vi "Run.vi"(8 "error in (no error)":errorcluster, 11 "Opctics in":refnum<class "Opt_Selector.lvclass">) -> (0 "error out":errorcluster, 3 "Opt_Selector out":refnum<class "Opt_Selector.lvclass">)   [LabVIEW 2018, in "Opt_Selector.lvclass"]
uses:
  Opt_Selector.lvclass
  Optics.lvclass/Optics.ctl
  Optics.lvclass
  StateMachine/State Machine.lvclass
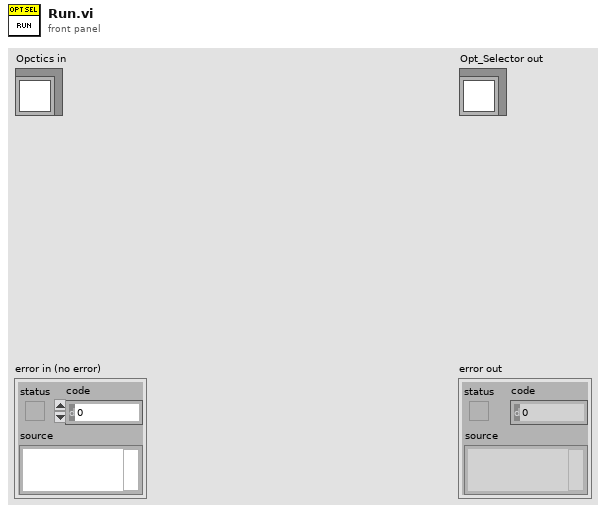
[diagram p1: front panel]
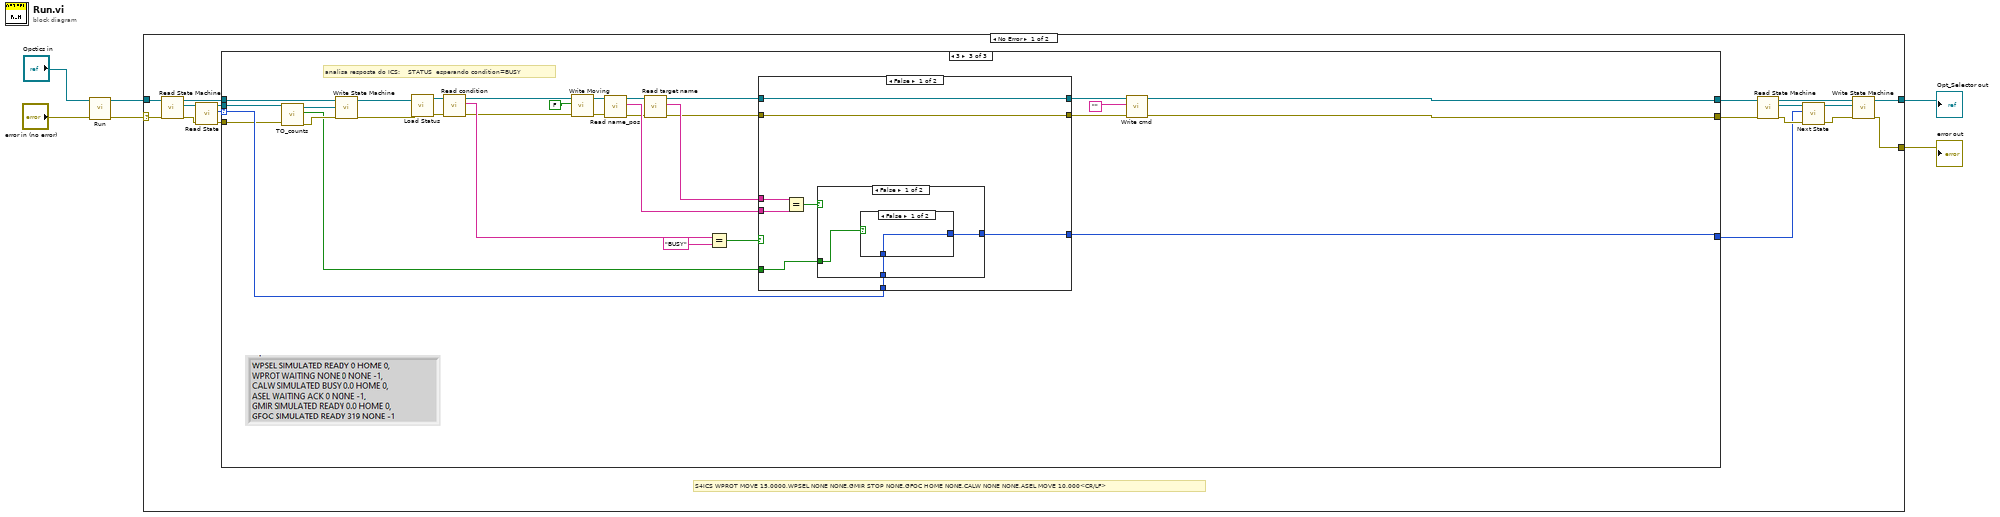
[diagram p0: block diagram]
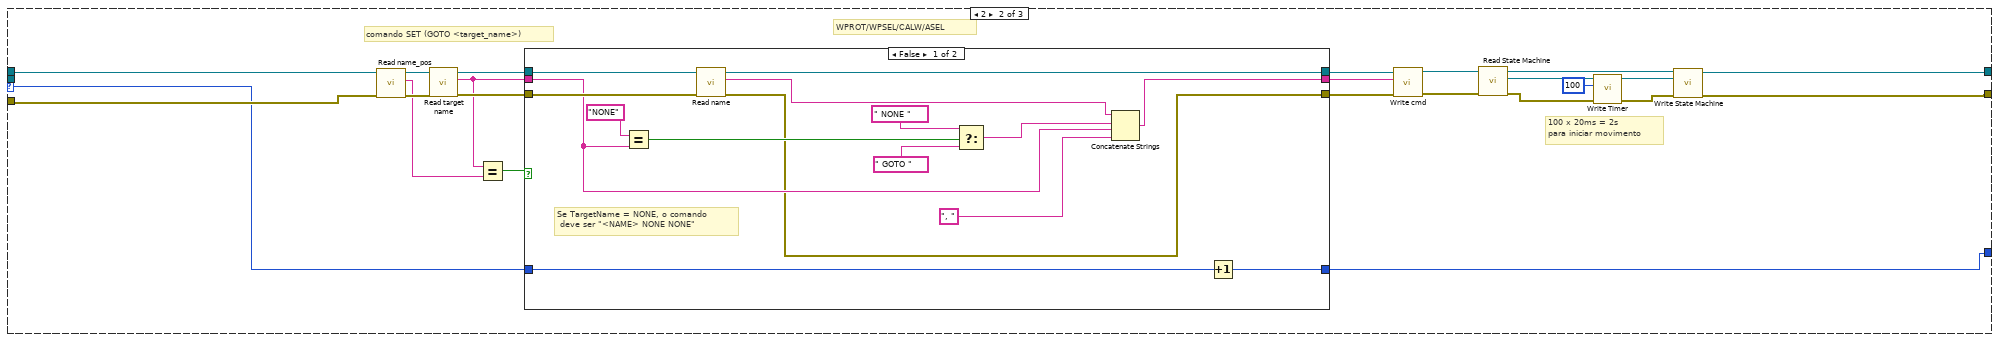
[diagram p3: hidden frame]
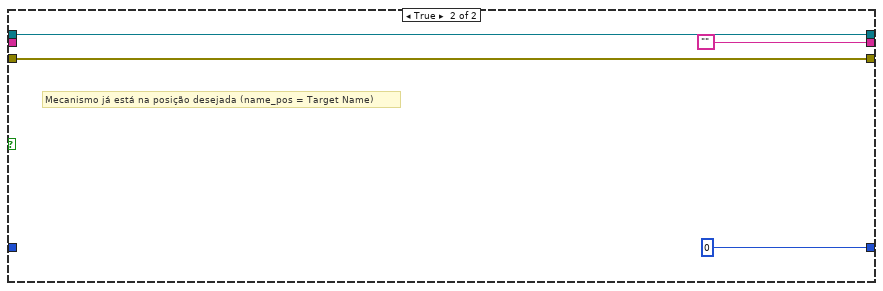
[diagram p4: hidden frame]
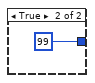
[diagram p5: hidden frame]
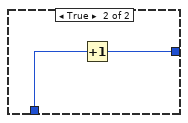
[diagram p6: hidden frame]
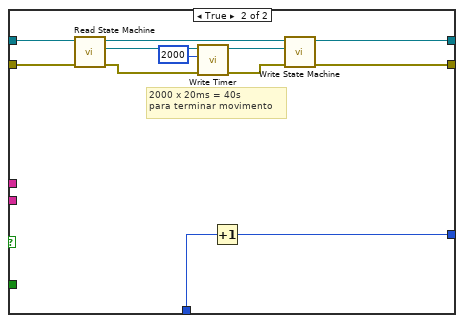
[diagram p7: hidden frame]
diagram:
  n1 = call-parent "Run.vi"("error in (no error)"="error in (no error)", "Opctics in"="Opctics in") -> ("error out"=w3:errorcluster, "Optics out"=w4:refnum<class "Opt_Selector.lvclass">)  [unwired: 8 in]
  n2 = case shown="No Error" w3 {
    selector: w3 -> [w23 w130]
    tunnel: [w8 w130] -> w1
    tunnel: [w13 w129] -> w2
    tunnel: w4 -> [w24 w129]
    frame No Error {
      # "S4ICS WPROT MOVE 15.0000,WPSEL NONE NONE,GMIR STOP NONE,GFOC HOME NONE,CALW NONE NONE,ASEL MOVE 10.000<CR/LF>"
      n3 = call-dynamic "Read State Machine.vi"("error in (no error)"=w23, "Device in"=w24) -> ("error out"=w20:errorcluster, "State Machine.lvclass"=w22:refnum<class "State Machine.lvclass">, "Device out"=w18:refnum<class "Opt_Selector.lvclass">)  [unwired: 7 in]
      n4 = call-dynamic "Read State.vi"("error in (no error)"=w20, "State Machine in"=w22) -> ("error out"=w19:errorcluster, "State"=w21:i32, "State Machine out"=w7:refnum<class "State Machine.lvclass">)  [unwired: 7 in]
      n5 = case shown="3" w21 {
        selector: w21 -> [w27 w45 w97]
        tunnel: w19 -> [w25 w48 w77]
        tunnel: [w25 w28 w99] -> w9
        tunnel: w18 -> [w26 w49 w80]
        tunnel: [w26 w29 w100] -> w16
        tunnel: [w27 w44 w98] -> w10
        tunnel: w7 -> [_ _ w76]
        frame Default {
        }
        frame 2 {
          # "100 x 20ms = 2s\npara iniciar movimento"
          # "WPROT/WPSEL/CALW/ASEL"
          # "comando SET (GOTO <target_name>)"
          n6 = call "Read name_pos.vi"("error in (no error)"=w48, "Optics in"=w49) -> ("error out"=w47:errorcluster, "name_pos"=w41:string, "Optics out"=w46:refnum<class "Opt_Selector.lvclass">)  [unwired: 7 in]
          n7 = call "Read target name.vi"("error in (no error)"=w47, "Optics in"=w46) -> ("error out"=w51:errorcluster, "target name"=w42:string, "Optics out"=w50:refnum<class "Opt_Selector.lvclass">)  [unwired: 7 in]
          n8 = Equal?(x=w42, y=w41) -> (x = y?=w43:bool)
          n9 = case shown="False" w43 {
            tunnel: [w54 w70] -> w40
            tunnel: [w53 w69] -> w39
            tunnel: w51 -> [w65 w69]
            tunnel: w50 -> [w64 w70]
            tunnel: w42 -> [w61 _]
            tunnel: w45 -> [w56 _]
            tunnel: [w55 0] -> w44
            tunnel: [w52 ""] -> w38
            frame False {
              # "Se TargetName = NONE, o comando\n deve ser \"<NAME> NONE NONE\""
              n10 = Equal?(x="NONE" ("y"), y=w61) -> (x = y?=w62:bool)
              n11 = call "Read name.vi"("error in (no error)"=w65, "Optics in"=w64) -> ("error out"=w53:errorcluster, "name"=w66:string, "Optics out"=w54:refnum<class "Opt_Selector.lvclass">)  [unwired: 7 in]
              n12 = Select(t=" NONE " ("string"), s=w62, f=" GOTO " ("string")) -> (s? t:f=w58:string)
              n13 = Concatenate Strings(w66, w58, w61, ", ") -> (w52:string)
              n14 = Increment(x=w56) -> (x+1=w55:i32)
            }
            frame True {
              # "Mecanismo já está na posição desejada (name_pos = Target Name)"
            }
          }
          n15 = call-dynamic "Write cmd.vi"("error in (no error)"=w39, "cmd"=w38, "Device in"=w40) -> ("error out"=w36:errorcluster, "Device out"=w35:refnum<class "Opt_Selector.lvclass">)  [unwired: 7 in]
          n16 = call-dynamic "Read State Machine.vi"("error in (no error)"=w36, "Device in"=w35) -> ("error out"=w31:errorcluster, "State Machine.lvclass"=w33:refnum<class "State Machine.lvclass">, "Device out"=w34:refnum<class "Opt_Selector.lvclass">)  [unwired: 7 in]
          n17 = call-dynamic "Write Timer.vi"("error in (no error)"=w31, "Timer"=u32 100, "State Machine in"=w33) -> ("error out"=w30:errorcluster, "State Machine out"=w32:refnum<class "State Machine.lvclass">)  [unwired: 7 in]
          n18 = call-dynamic "Write State Machine.vi"("error in (no error)"=w30, "State Machine.lvclass"=w32, "Device in"=w34) -> ("error out"=w28:errorcluster, "Device out"=w29:refnum<class "Opt_Selector.lvclass">)  [unwired: 7 in]
        }
        frame 3 {
          # "analisa resposta do ICS:    STATUS  esperando condition=BUSY"
          n19 = call-dynamic "TO_counts.vi"("error in (no error)"=w77, "State Machine in"=w76) -> ("error out"=w81:errorcluster, "timer zero"=w75:bool, "State Machine out"=w82:refnum<class "State Machine.lvclass">)  [unwired: 7 in]
          n20 = call-dynamic "Write State Machine.vi"("error in (no error)"=w81, "State Machine.lvclass"=w82, "Device in"=w80) -> ("error out"=w78:errorcluster, "Device out"=w79:refnum<class "Opt_Selector.lvclass">)  [unwired: 7 in]
          n21 = call-dynamic "Load Status.vi"("error in (no error)"=w78, "Optics in"=w79) -> ("error out"=w86:errorcluster, "Optics out"=w85:refnum<class "Opt_Selector.lvclass">)  [unwired: 8 in]
          n22 = call "Read condition.vi"("error in (no error)"=w86, "Optics in"=w85) -> ("error out"=w83:errorcluster, "condition"=w87:string, "Optics out"=w84:refnum<class "Opt_Selector.lvclass">)  [unwired: 7 in]
          n23 = call-dynamic "Write Moving.vi"("error in (no error)"=w83, "Moving"=FALSE, "Optics in"=w84) -> ("error out"=w88:errorcluster, "Optics out"=w89:refnum<class "Opt_Selector.lvclass">)  [unwired: 7 in]
          n24 = call "Read name_pos.vi"("error in (no error)"=w88, "Optics in"=w89) -> ("error out"=w91:errorcluster, "name_pos"=w92:string, "Optics out"=w90:refnum<class "Opt_Selector.lvclass">)  [unwired: 7 in]
          n25 = call "Read target name.vi"("error in (no error)"=w91, "Optics in"=w90) -> ("error out"=w72:errorcluster, "target name"=w94:string, "Optics out"=w74:refnum<class "Opt_Selector.lvclass">)  [unwired: 7 in]
          n26 = Equal?(x=w87, y="BUSY") -> (x = y?=w95:bool)
          n27 = case shown="False" w95 {
            tunnel: [w106 w127] -> w98
            tunnel: w97 -> [w107 w128]
            tunnel: w94 -> [w109 _]
            tunnel: w92 -> [w108 _]
            tunnel: w75 -> [w104 _]
            tunnel: [w103 w118] -> w73
            tunnel: w74 -> [w103 w120]
            tunnel: [w102 w117] -> w71
            tunnel: w72 -> [w102 w119]
            frame False {
              n28 = Equal?(x=w109, y=w108) -> (x = y?=w105:bool)
              n29 = case shown="False" w105 {
                tunnel: [w111 w116] -> w106
                tunnel: w107 -> [w110 w115]
                tunnel: w104 -> [w112 _]
                frame False {
                  n30 = case shown="False" w112 {
                    tunnel: [w113 99] -> w111
                    tunnel: w110 -> [w113 _]
                    frame False {
                    }
                    frame True {
                    }
                  }
                }
                frame True {
                  n31 = Increment(x=w115) -> (x+1=w116:i32)
                }
              }
            }
            frame True {
              # "2000 x 20ms = 40s\npara terminar movimento"
              n32 = call-dynamic "Read State Machine.vi"("error in (no error)"=w119, "Device in"=w120) -> ("error out"=w122:errorcluster, "State Machine.lvclass"=w124:refnum<class "State Machine.lvclass">, "Device out"=w125:refnum<class "Opt_Selector.lvclass">)  [unwired: 7 in]
              n33 = call-dynamic "Write Timer.vi"("error in (no error)"=w122, "Timer"=u32 2000, "State Machine in"=w124) -> ("error out"=w121:errorcluster, "State Machine out"=w123:refnum<class "State Machine.lvclass">)  [unwired: 7 in]
              n34 = Increment(x=w128) -> (x+1=w127:i32)
              n35 = call-dynamic "Write State Machine.vi"("error in (no error)"=w121, "State Machine.lvclass"=w123, "Device in"=w125) -> ("error out"=w117:errorcluster, "Device out"=w118:refnum<class "Opt_Selector.lvclass">)  [unwired: 7 in]
            }
          }
          n36 = call-dynamic "Write cmd.vi"("error in (no error)"=w71, "cmd"="", "Device in"=w73) -> ("error out"=w99:errorcluster, "Device out"=w100:refnum<class "Opt_Selector.lvclass">)  [unwired: 7 in]
        }
      }
      n37 = call-dynamic "Read State Machine.vi"("error in (no error)"=w9, "Device in"=w16) -> ("error out"=w12:errorcluster, "State Machine.lvclass"=w15:refnum<class "State Machine.lvclass">, "Device out"=w14:refnum<class "Opt_Selector.lvclass">)  [unwired: 7 in]
      n38 = call "Next State.vi"("error in (no error)"=w12, "New_State"=w10, "State Machine in"=w15) -> ("error out"=w11:errorcluster, "State Machine out"=w17:refnum<class "State Machine.lvclass">)  [unwired: 7 in]
      n39 = call-dynamic "Write State Machine.vi"("error in (no error)"=w11, "State Machine.lvclass"=w17, "Device in"=w14) -> ("error out"=w8:errorcluster, "Device out"=w13:refnum<class "Opt_Selector.lvclass">)  [unwired: 7 in]
    }
    frame Error {
    }
  }
  "error out" <- w1
  "Opt_Selector out" <- w2
